vi "Login.vi"(0 "User Manager Model in":refnum<class "User Manager Model.lvclass">, 5 "Credentials":T1, 11 "error in (no error)":errorcluster) -> (4 "User Manager Model out":refnum<class "User Manager Model.lvclass">, 15 "error out":errorcluster)   [LabVIEW 2020, in "User Manager Model.lvlib" / "User Manager Model.lvclass"]
uses:
  <vilib>/gpm_packages/@cs/User Manager App/User Manager Model/User Manager Model/User Manager Model.lvclass
  C:/Program Files/National Instruments/LabVIEW 2020/vi.lib/gpm_packages/@cs/mva-core/Source/IModel/IModel/IModel.lvclass
  <vilib>/gpm_packages/@cs/User Manager App/User Manager Model/Type Definitions/Credentials.ctl
  <vilib>/gpm_packages/@cs/user-manager/Source/User Configuration Manager/User Configuration Manager.lvclass
  C:/Program Files/National Instruments/LabVIEW 2020/vi.lib/gpm_packages/@cs/user-manager/Source/iUser Configuration Manager/iUser Configuration Manager.lvclass
  <vilib>/gpm_packages/@cs/User Manager App/User Manager Model/User Manager Model/User Manager Model.lvclass/User Manager Model.ctl
  <vilib>/gpm_packages/@cs/persistence/source/XML/XML.lvclass
  C:/Program Files/National Instruments/LabVIEW 2020/vi.lib/gpm_packages/@cs/persistence/source/IPersist/IPersist.lvclass
  <vilib>/gpm_packages/@cs/mva-core/Source/IObserver/IObserver/IObserver.lvclass/IObserver.ctl
  <vilib>/gpm_packages/@cs/mva-core/Source/IModel/IModel/IModel.lvclass/IModel.ctl
  <vilib>/gpm_packages/@cs/mva-core/Source/IMediator/PublishRequest/PublishRequest.lvclass/PublishRequest.ctl
  <vilib>/gpm_packages/@cs/mva-core/Source/IMediator/IMediator Messages/Publish Msg/Publish Msg.lvclass/Publish Msg.ctl
  <vilib>/gpm_packages/@cs/actor-framework-messages/Source/RoundTripMessage/RoundTripMessage.lvclass/RoundTripMessage.ctl
  <vilib>/ActorFramework/Message Enqueuer/Message Enqueuer.lvclass/Message Enqueuer.ctl
  <vilib>/gpm_packages/@cs/User Manager App/User Manager Model/Type Definitions/Successful Login Information.ctl
  <vilib>/gpm_packages/@cs/User Manager App/User Manager Model/Type Definitions/User Levels.ctl
  <vilib>/gpm_packages/@cs/User Manager App/User Manager Model/User Manager Model/Accessors/Read Persistence Path.vi
  <vilib>/gpm_packages/@cs/mva-core/Source/IMediator/IMediator Messages/Publish Msg/Send Pre-Addressed Publish.vi
  <vilib>/gpm_packages/@cs/mva-core/Source/IObserver/IObserver/Read Unique ID.vi
  <vilib>/gpm_packages/@cs/mva-core/Source/IMediator/PublishRequest/Pack Publish Request.vi
  <vilib>/gpm_packages/@cs/actor-framework-messages/Source/RoundTripMessage/Return Round-Trip Message.vi
  <vilib>/ActorFramework/Message Enqueuer/Enqueue.vi
  <vilib>/gpm_packages/@cs/mva-core/Source/IModel/IModel/IModel.lvclass
  C:/Program Files/National Instruments/LabVIEW 2020/vi.lib/gpm_packages/@cs/mva-core/Source/IObserver/IObserver/IObserver.lvclass
  <vilib>/gpm_packages/@cs/mva-core/Source/IMediator/IMediator Messages/Publish Msg/Publish Msg.lvclass
  C:/Program Files/National Instruments/LabVIEW 2020/vi.lib/gpm_packages/@cs/actor-framework-messages/Source/RoundTripMessage/RoundTripMessage.lvclass
  <vilib>/gpm_packages/@cs/actor-framework-messages/Source/RoundTripMessage/RoundTripMessage.lvclass
  C:/Program Files/National Instruments/LabVIEW 2020/vi.lib/ActorFramework/Message/Message.lvclass
  <vilib>/Utility/error.llb/Error Cluster From Error Code.vi
  <vilib>/ActorFramework/Message Priority Queue/Priority Enqueue.vi
  <vilib>/gpm_packages/@cs/mva-core/Source/IMediator/PublishRequest/PublishRequest.lvclass
  <vilib>/gpm_packages/@cs/user-manager/Source/User Configuration Manager Ref/By Ref.lvlib
  <vilib>/gpm_packages/@cs/User Manager App/User Manager Model/Type Definitions/User Manager Application Types.lvlib
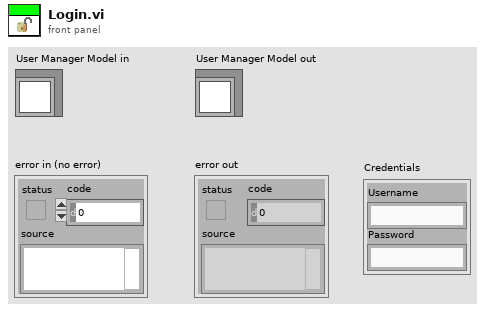
[diagram p1: front panel]
types:
  T1 = typedef "User Manager Application Types.lvlib/Credentials.ctl" = cluster{"Username":string, "Password":string}
  T2 = typedef "User Manager Application Types.lvlib/User Levels.ctl" = cluster{"Rank":i32, "Title":string}
  T3 = typedef "User Manager Application Types.lvlib/Successful Login Information.ctl" = cluster{"Username":string, "User Level":T2, "User Levels In This Society":T2[]}
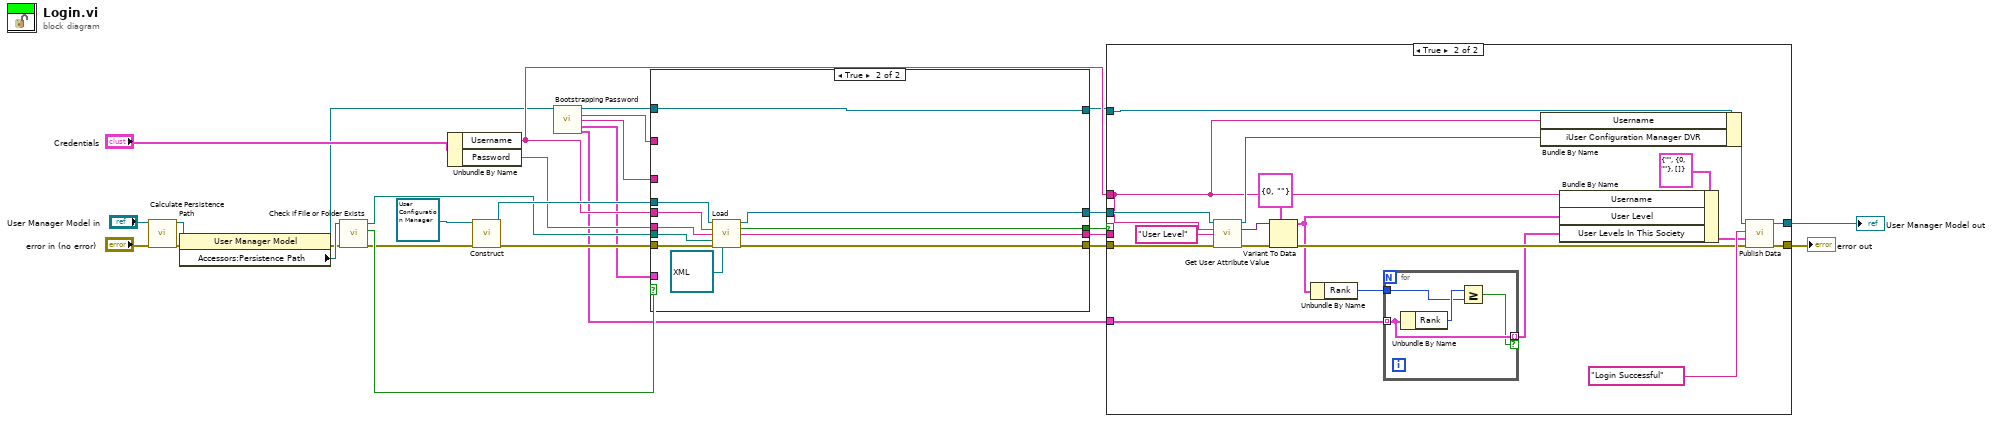
[diagram p0: block diagram]
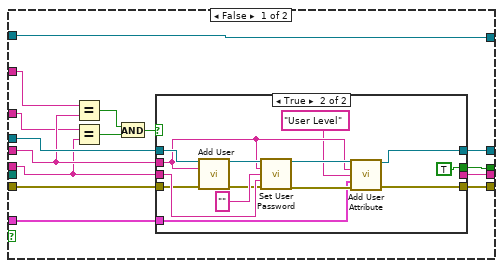
[diagram p2: hidden frame]
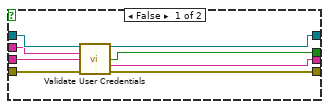
[diagram p3: hidden frame]
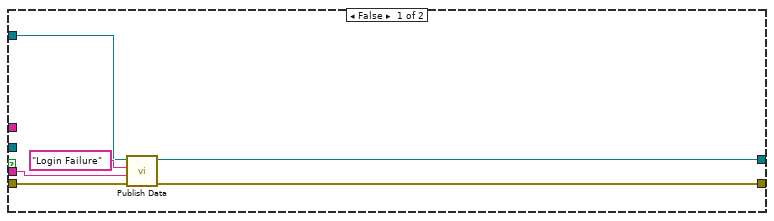
[diagram p4: hidden frame]
diagram:
  n1 = call-dynamic "Calculate Persistence Path.vi"("User Manager Model in"="User Manager Model in", "error in (no error)"="error in (no error)") -> ("User Manager Model out"=w13:refnum<class "User Manager Model.lvclass">, "error out"=w8:errorcluster)  [unwired: 12 in]
  n2 = property on="Property Node" class="User Manager Model"(reference=w13, error in=w8) -> (reference out=w11:refnum<class "User Manager Model.lvclass">, error out=w9:errorcluster, "Accessors:Persistence Path"=w10:path)
  n3 = call <vilib>:"Check if File or Folder Exists.vi"("error in (no error)"=w9, "path"=w10) -> ("error out"=w7:errorcluster, "file or folder exists?"=w17:bool, "dup path"=w16:path)  [unwired: 7 in]
  n4 = Unbundle By Name("Credentials") -> ("Username"=w15:string, "Password"=w23:string)
  n5 = call <vilib>:"Construct.vi"("iUser Configuration Manager in"=refnum<class "User Configuration Manager.lvclass"> refnum ("User Configuration Manager.lvlib:User Configuration Manager"), "error in"=w7) -> ("dup iUser Configuration Manager DVR"=w25:refnum<data-value>, "error out"=w20:errorcluster)  [unwired: 12 in]
  n6 = call-dynamic "Bootstrapping Password.vi"("User Manager Model in"=w11) -> ("User Manager Model out"=w2:refnum<class "User Manager Model.lvclass">, "Username"=w6:string, "Password"=w5:string, "User Level"=w4:T2, "User Levels In This Society"=w3:T2[])  [unwired: 10 in]
  n7 = case shown="True" w17 {
    tunnel: w25 -> [w43 w72]
    tunnel: w15 -> [w35 w76]
    tunnel: w23 -> [w34 w67]
    tunnel: [w39 w74] -> w22
    tunnel: [w42 w75] -> w21
    tunnel: w20 -> [w33 w71]
    tunnel: [w41 w73] -> w19
    tunnel: [w40 w70] -> w18
    tunnel: w16 -> [_ w68]
    tunnel: [w29 w66] -> w1
    tunnel: w2 -> [w29 w66]
    tunnel: w6 -> [w32 _]
    tunnel: w5 -> [w31 _]
    tunnel: w4 -> [w30 _]
    frame False {
      n8 = Equal?(x=w32, y=w35) -> (x = y?=w37:bool)
      n9 = Equal?(x=w31, y=w34) -> (x = y?=w36:bool)
      n10 = And(x=w37, y=w36) -> (x .and. y?=w38:bool)
      n11 = case shown="True" w38 {
        tunnel: w43 -> [w51 w64]
        tunnel: w35 -> [w50 w54]
        tunnel: w34 -> [w49 w62]
        tunnel: [w48 _] -> w42
        tunnel: w33 -> [w47 w60]
        tunnel: [w46 w56] -> w41
        tunnel: [w45 w55] -> w40
        tunnel: [w44 TRUE] -> w39
        tunnel: w30 -> [_ w52]
        frame False {
          n12 = call <vilib>:"Validate User Credentials.vi"("iUser Configuration Manager DVR"=w51, "Username"=w50, "Password"=w49, "error in"=w47) -> ("dup iUser Configuration Manager DVR"=w46:refnum<data-value>, "Verified"=w44:bool, "Verification Message"=w48:string, "error out"=w45:errorcluster)  [unwired: 7 in, 1 out]
        }
        frame True {
          n13 = call <vilib>:"Add User.vi"("iUser Configuration Manager DVR"=w64, "Username"=w54, "error in"=w60) -> ("dup iUser Configuration Manager DVR"=w63:refnum<data-value>, "error out"=w59:errorcluster)  [unwired: 10 in, 1 out]
          n14 = call <vilib>:"Set User Password.vi"("iUser Configuration Manager DVR"=w63, "Username"=w54, "Current Password"="", "New Password"=w62, "error in"=w59) -> ("dup iUser Configuration Manager DVR"=w58:refnum<data-value>, "error out"=w57:errorcluster)  [unwired: 8 in, 1 out]
          n15 = call <vilib>:"Add User Attribute.vi"("iUser Configuration Manager DVR"=w58, "Username"=w54, "Attribute Name"="User Level", "Attribute Value"=w52, "error in"=w57) -> ("dup iUser Configuration Manager DVR"=w56:refnum<data-value>, "error out"=w55:errorcluster)  [unwired: 8 in, 1 out]
        }
      }
    }
    frame True {
      n16 = call <vilib>:"Load.vi"("iUser Configuration Manager DVR"=w72, "Username"=w76, "Password"=w67, "Path"=w68, "error in"=w71, "Persistence"=refnum<class "XML.lvclass"> refnum ("XML.lvlib:XML.lvclass")) -> ("dup iUser Configuration Manager DVR"=w73:refnum<data-value>, "Verified"=w74:bool, "Verification Message"=w75:string, "error out"=w70:errorcluster)  [unwired: 6 in]
    }
  }
  n17 = case shown="True" w22 {
    tunnel: [w82 w101] -> w28
    tunnel: [w80 w100] -> w27
    tunnel: w21 -> [w77 _]
    tunnel: w1 -> [w79 w99]
    tunnel: w19 -> [_ w95]
    tunnel: w18 -> [w78 w93]
    tunnel: w15 -> [_ w87]
    tunnel: w3 -> [_ w84]
    frame False {
      n18 = call <vilib>:"Publish Data.vi"("error in (no error)"=w78, "Data to Publish"=w77, "Datum Name"="Login Failure", "IModel in"=w79) -> ("error out"=w80:errorcluster, "IModel out"=w82:refnum<class "User Manager Model.lvclass">)  [unwired: 6 in]
    }
    frame True {
      n19 = call <vilib>:"Get User Attribute Value.vi"("iUser Configuration Manager DVR"=w95, "Username"=w87, "Attribute Name"="User Level", "error in"=w93) -> ("dup iUser Configuration Manager DVR"=w94:refnum<data-value>, "Attribute Value"=w91:variant, "error out"=w90:errorcluster)  [unwired: 8 in, 1 out]
      n20 = Variant To Data(error in=w90, type=T2 {"Rank"=0, "Title"=""} ("User Level"), Variant=w91) -> (data=w86:T2, error out=w89:errorcluster)
      n21 = Unbundle By Name(w86) -> ("Rank"=w85:i32)
      n22 = for {
        tunnel: w85 -> [w104]
        tunnel: w84 -> [w106] mode=indexing
        tunnel: [w106] -> w83 mode=indexing if=w103
        n23 = Unbundle By Name(w106) -> ("Rank"=w105:i32)
        n24 = Greater Or Equal?(x=w105, y=w104) -> (x >= y?=w103:bool)
      }
      n25 = Bundle By Name(cluster=w99, "Username"=w87, "iUser Configuration Manager DVR"=w94) -> (w98:refnum<class "User Manager Model.lvclass">)
      n26 = Bundle By Name(cluster=T3 {"Username"="", "User Level"={"Rank"=0, "Title"=""}, "User Levels In This Society"=[]}, "Username"=w87, "User Level"=w86, "User Levels In This Society"=w83) -> (w96:T3)
      n27 = call <vilib>:"Publish Data.vi"("error in (no error)"=w89, "Data to Publish"=w96, "Datum Name"="Login Successful", "IModel in"=w98) -> ("error out"=w100:errorcluster, "IModel out"=w101:refnum<class "User Manager Model.lvclass">)  [unwired: 6 in]
    }
  }
  "error out" <- w27
  "User Manager Model out" <- w28
